vi "Q8381 RESOLUTION.vi"(2 "resolution":u16(ring) items=["0.1 nm", "0.2 nm", "0.5 nm", "1.0 nm", "2.0 nm", "5.0 nm"], 3 "GPIB Address":u16=8 max=31 step=1, 4 "VISA resource name":refnum<visa-resource-name>) -> (0 "GPIB Status":bool, 1 "UNCAL":bool)   [LabVIEW 2017]
doc: "resolution:\n 0: 0.1nm, 1: 0.2nm,\n 2: 0.5nm, 3: 1.0nm,\n 4: 2.0nm, 5: 5.0nm."
panel:
  out "Numeric 2":dbl
  out "R>=":dbl
  out "Value":string
  out "Power":string
  out "read buffer":string
  out "Numeric":string
  out "Program Code":string
  # "RESOLUTION"
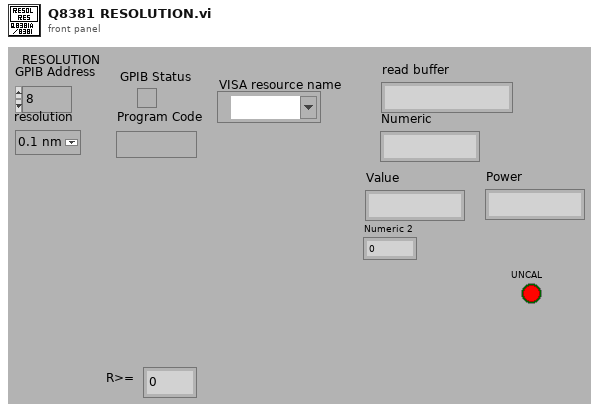
[diagram p1: front panel]
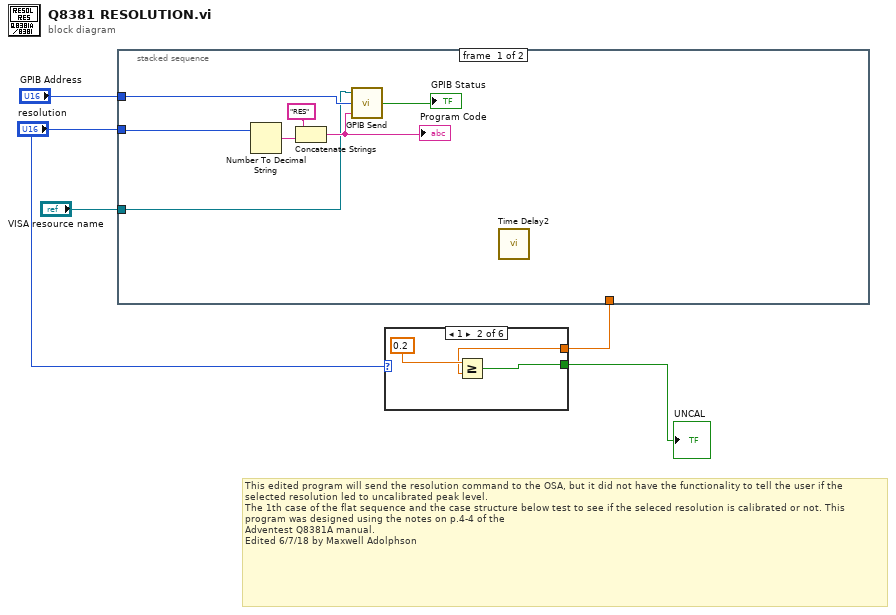
[diagram p0: block diagram]
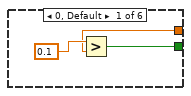
[diagram p2: hidden frame]
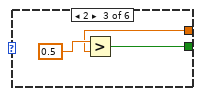
[diagram p3: hidden frame]
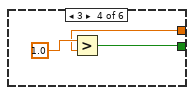
[diagram p4: hidden frame]
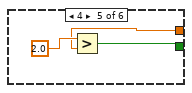
[diagram p5: hidden frame]
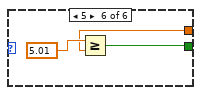
[diagram p6: hidden frame]
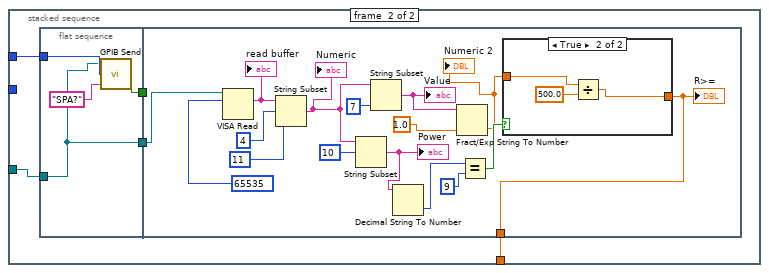
[diagram p7: hidden frame]
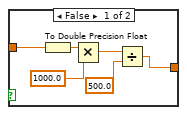
[diagram p8: hidden frame]
diagram:
  # "This edited program will send the resolution command to the OSA, but it did not have the functionality to tell the user if the selected resolution led to uncalibrated peak level. \nThe 1th case of the flat sequence and the case structure below test to see if the seleced resolution is calibrated or not. This program was designed using the notes on p.4-4 of the \nAdventest Q8381A manual.\nEdited 6/7/18 by Maxwell Adolphson"
  n1 = stacked-sequence {
    tunnel: "resolution" -> [w12 _]
    tunnel: "GPIB Address" -> [w8 w14]
    tunnel: "VISA resource name" -> [w6 w17]
    tunnel: [_ w15] -> w1
    frame #0 {
      n2 = Number To Decimal String(number=w12) -> (decimal integer string=w11:string)  [unwired: 1 in]
      n3 = Concatenate Strings("RES", w11) -> (w9:string)
      "Program Code" <- w9
      n4 = call "GPIB Send.vi"("Command String"=w9, "Address"=w8, "VISA resource name"=w6) -> ("Error"=→"GPIB Status":bool)
      n5 = call "Time Delay2"() -> ()  [unwired: 11 in, 1 out]
    }
    frame #1 {
      n6 = flat-sequence {
        tunnel: w17 -> [w18]
        tunnel: [w21] -> w16
        tunnel: w14 -> [w19]
        tunnel: [w18] -> w13
        tunnel: w16 -> [_]
        tunnel: [w23] -> w15
        tunnel: w13 -> [w22]
        frame #0 {
          n7 = call "GPIB Send.vi"("Command String"="SPA?" ("write buffer"), "Address"=w19, "VISA resource name"=w18) -> ("Error"=w21:bool)
        }
        frame #1 {
          n8 = VISA Read(VISA resource name=w22, byte count=u32 65535) -> (read buffer=w34:string)  [unwired: 1 in, 3 out]
          "read buffer" <- w34
          n9 = String Subset(string=w34, offset (0)=4, length (rest)=11 ("length (rest)")) -> (substring=w32:string)
          "Numeric" <- w32
          n10 = String Subset(string=w32, offset (0)=10) -> (substring=w30:string)  [unwired: 1 in]
          "Power" <- w30
          n11 = String Subset(string=w32, length (rest)=7 ("length (rest)")) -> (substring=w27:string)  [unwired: 1 in]
          "Value" <- w27
          n12 = Decimal String To Number(string=w30) -> (number=w24:i32)  [unwired: 2 in, 1 out]
          n13 = Fract/Exp String To Number(string=w27, default (0 dbl)=1.0) -> (number=w26:dbl)  [unwired: 2 in, 1 out]
          "Numeric 2" <- w26
          n14 = Equal?(x=w24, y=9) -> (x = y?=w28:bool)
          n15 = case shown="True" w28 {
            tunnel: [w38 w46] -> w23
            tunnel: w26 -> [w41 w45]
            frame False {
              n16 = To Double Precision Float(number=w41) -> (double precision float=w42:dbl)
              n17 = Multiply(x=w42, y=1000.0) -> (x*y=w40:dbl)
              n18 = Divide(x=w40, y=500.0) -> (x/y=w38:dbl)
            }
            frame True {
              n19 = Divide(x=w45, y=500.0) -> (x/y=w46:dbl)
            }
          }
          "R>=" <- w23
        }
      }
    }
  }
  n20 = case shown="1" "resolution" {
    tunnel: [w48 w51 w54 w57 w60 w63] -> w2
    tunnel: w1 -> [w47 w50 w53 w56 w59 w62]
    frame 0, Default {
      n21 = Greater?(x=0.1, y=w47) -> (0:w48:bool)
    }
    frame 1 {
      n22 = Greater Or Equal?(x=0.2, y=w50) -> (x >= y?=w51:bool)
    }
    frame 2 {
      n23 = Greater?(x=0.5, y=w53) -> (0:w54:bool)
    }
    frame 3 {
      n24 = Greater?(x=1.0, y=w56) -> (0:w57:bool)
    }
    frame 4 {
      n25 = Greater?(x=2.0, y=w59) -> (0:w60:bool)
    }
    frame 5 {
      n26 = Greater Or Equal?(x=5.01, y=w62) -> (x >= y?=w63:bool)
    }
  }
  "UNCAL" <- w2
